vi "Get Joystick Button Configuration.vi"(7 "Event Type (1: pressed)":i32(ring)=1 items=["pressed"=1, "released before 1 second"=2, "held for 1 second"=3, "released after 1 second"=4], 8 "error in (no error)":errorcluster, 9 "Joystick Device Number":string, 10 "Key Index (1)":u8=1, 11 "VISA resource name":refnum<visa-resource-name>) -> (0 "error out":errorcluster, 2 "Command List":string[](array[string]), 3 "VISA resource name out":refnum<visa-resource-name>)   [LabVIEW 2018, in "Zaber A Series.lvlib"]
doc: "Use this VI to find out what commands are associated with a key event on a joystick.\n\nYou must specify the device number of the joystick and the index of the key to check. Different models of joystick may have different numbers of keys.\n\nYou should also select the specific key event that you want to fire the commands. Different lists of commands can be triggered by each of four key events: initial press (1), release after less than a second (2), hold for a second or more (3), and release after a second (4).\n\nThe output will be an array of commands that the joystick will generate when the specified key event occurs, or an empty array if there are none.\n\nThis VI expects the serial port to already have been configured."
uses:
  Zaber A Series.lvlib
  Private/All Commands.ctl
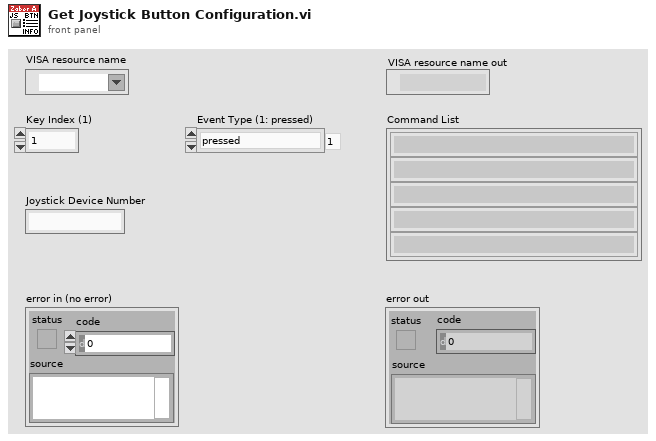
[diagram p1: front panel]
types:
  T1 = typedef "Zaber A Series.lvlib/All Commands.ctl" = string
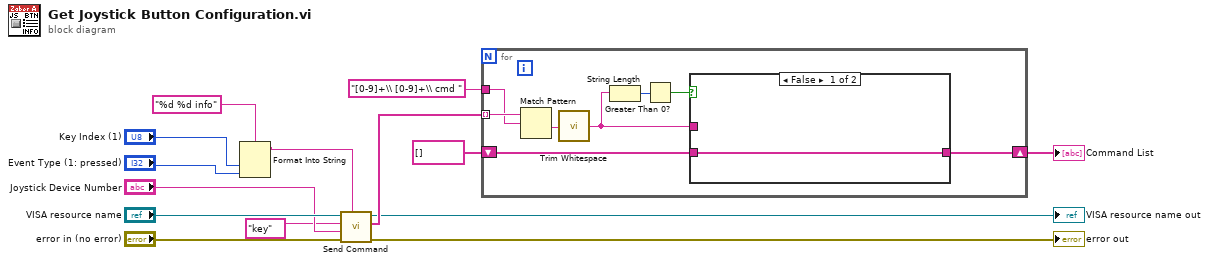
[diagram p0: block diagram]
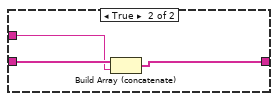
[diagram p2: hidden frame]
diagram:
  n1 = Format Into String(format string="%d %d info", "Key Index (1)", "Event Type (1: pressed)") -> (resulting string=w6:string)  [unwired: 2 in, 1 out]
  n2 = call "Send Command.vi"("Data"=w6, "error in (no error)"="error in (no error)", "Device and Axis"="Joystick Device Number", "Command"=T1 "key" ("Complete Command List"), "VISA resource name"="VISA resource name") -> ("error out"=→"error out":errorcluster, "Response String Array"=w9:string[], "VISA resource name out"=→"VISA resource name out":refnum<visa-resource-name>)  [unwired: 1 in, 3 out]
  n3 = for {
    shift-right: [w16] -> w10
    shift-left: string[] [] -> [w17]
    tunnel: w9 -> [w22] mode=indexing
    tunnel: "[0-9]+\\ [0-9]+\\ cmd " ("regular expression") -> [w19]
    n4 = Match Pattern(string=w22, regular expression=w19) -> (after substring=w21:string)  [unwired: 1 in, 3 out]
    n5 = call <vilib>:"Trim Whitespace.vi"("string"=w21) -> ("trimmed string"=w15:string)  [unwired: 1 in]
    n6 = String Length(string=w15) -> (length=w20:i32)
    n7 = Greater Than 0?(x=w20) -> (x > 0?=w18:bool)
    n8 = case shown="False" w18 {
      tunnel: w17 -> [w23 w26]
      tunnel: [w23 w25] -> w16
      tunnel: w15 -> [_ w24]
      frame False {
      }
      frame True {
        n9 = Build Array (concatenate)(w26, w24) -> (w25:string[])
      }
    }
  }
  "Command List" <- w10
